vi "Enqueue - Delayed.vi"(8 "error in (no error)":errorcluster, 9 "Delay Time (ms)":i32=1000, 10 "Command":string, 11 "Queue with Cluster Reference":T1) -> (0 "error out":errorcluster, 3 "Queue Out (dup)":T1)   [LabVIEW 2010]
doc: "This VI enqueues a command to handle delayed timing. The item is sent to the \"State - Delayed Insert\" case (must be handled in your state machine) with the first argument being the command to enqueue after the delay. The timer VI is reset to permit using it to determine if time has expired. Delay Time is enqueued as the data.\n\nInputs:\nQueue with Cluster Reference - (queue) queue to insert cluster into\nCommand - (string) command to be inserted after the delay time has expired\nDelay Time (ms) - (I32) time to wait before enqueuing the command\nerror in - error input cluster\n\nOutputs:\nQueue Out (dup) - (queue) duplicate reference to input queue\nerror out - error output cluster"
uses:
  <userlib>/Common/Queue with Cluster/TYP_Queue with Cluster Reference.ctl
panel:
  # "Inputs"
  # "Outputs"
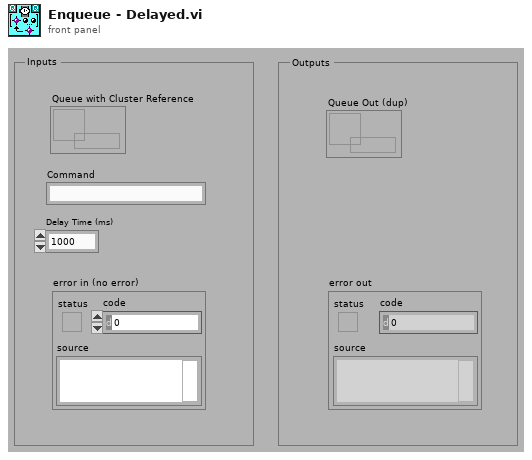
[diagram p1: front panel]
types:
  T1 = typedef "TYP_Queue with Cluster Reference.ctl" = refnum<queue>
  T2 = typedef "TYP_Queue Cluster Element.ctl" = cluster{"Command":string, "Data":variant}
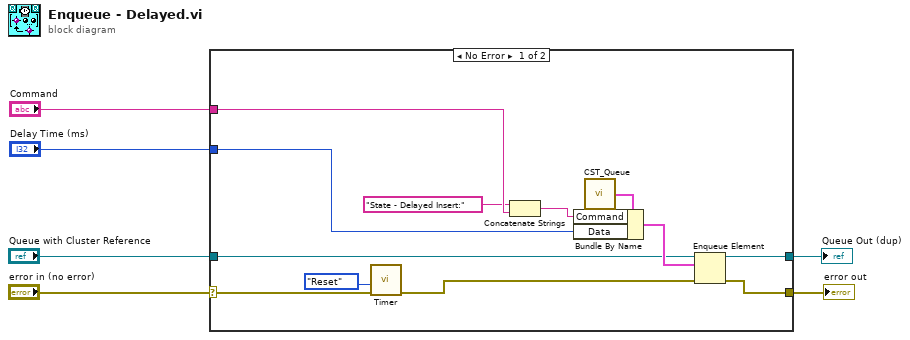
[diagram p0: block diagram]
diagram:
  n1 = case shown="No Error" "error in (no error)" {
    selector: "error in (no error)" -> [w14 w20]
    tunnel: [w15 w20] -> w5
    tunnel: "Command" -> [w10 _]
    tunnel: "Delay Time (ms)" -> [w7 _]
    tunnel: "Queue with Cluster Reference" -> [w16 w19]
    tunnel: [w8 w19] -> w1
    frame No Error {
      n2 = call <userlib>:"Timer.vi"("error in (no error)"=w14, "Command"=enum16{"Reset", "Get Time", "Check Time"}."Reset") -> ("error out"=w13:errorcluster)  [unwired: 7 in, 2 out]
      n3 = Concatenate Strings("State - Delayed Insert:" ("Command"), w10) -> (w11:string)
      n4 = call <userlib>:"CST_Queue.vi"() -> ("Queue Cluster Element"=w18:T2)  [unwired: 1 in]
      n5 = Bundle By Name(cluster=w18, "Command"=w11, "Data"=w7) -> (w17:T2)
      n6 = Enqueue Element(queue=w16, element=w17, error in (no error)=w13) -> (queue out=w8:T1, error out=w15:errorcluster)  [unwired: 1 in, 1 out]
    }
    frame Error {
    }
  }
  "error out" <- w5
  "Queue Out (dup)" <- w1
